vi "Make Panel Draggable - Drop In.vi"(0 "User Event":refnum<user-event>, 11 "error in (no error)":errorcluster) -> (15 "error out":errorcluster)   [LabVIEW 2011]
uses:
  <vilib>/Utility/inputDevices.llb/mouseAcquire.vi
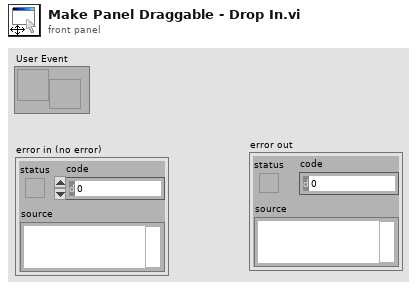
[diagram p1: front panel]
types:
  T1 = cluster{"Event Registration Refnum":refnum<event-registration>, "Event Registration Refnum":refnum<event-registration>}
  T2 = cluster{"Horizontal":i32, "Vertical":i32, "Scrolling":i32}
  T3 = typedef "LVRectTypeDef.ctl" = cluster{"left":i16, "top":i16, "right":i16, "bottom":i16}
  T4 = cluster{"button 1":bool, "button 2":bool, "button 3":bool, "button 4":bool}
  T5 = cluster{"Horizontal":i32, "Vertical":i32, "Horizontal":i32, "Vertical":i32}
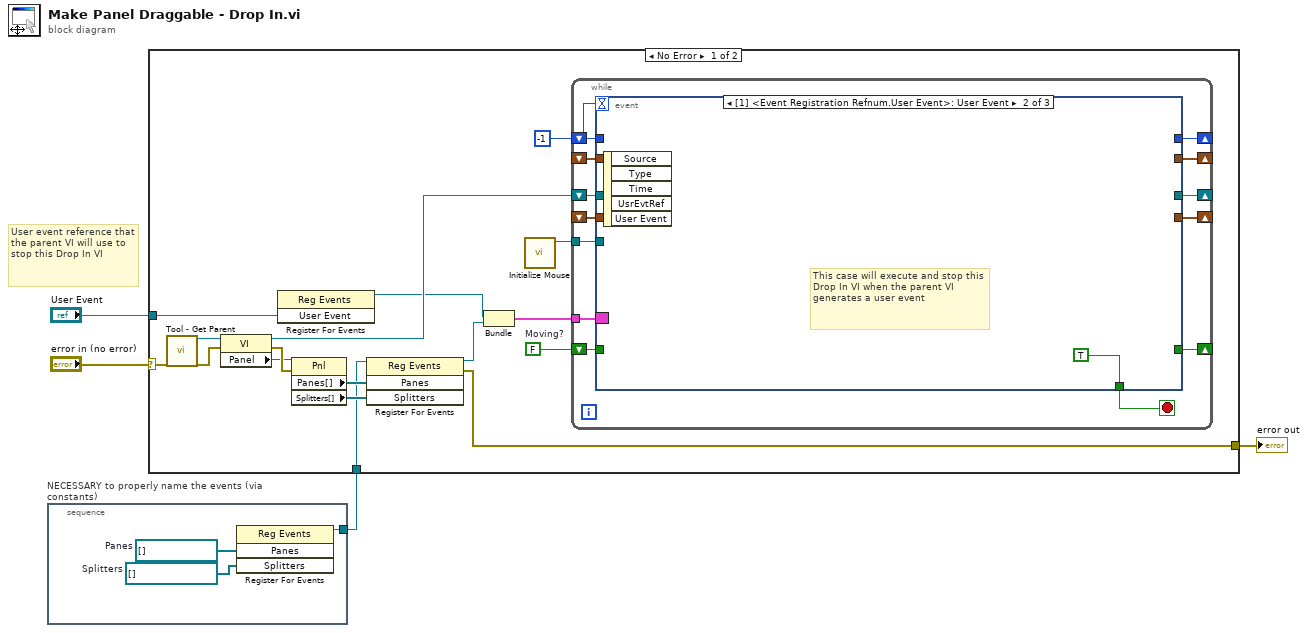
[diagram p0: block diagram]
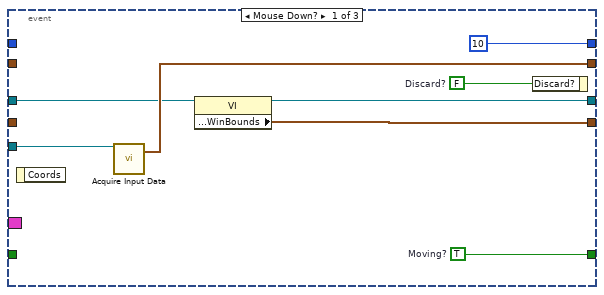
[diagram p2: hidden frame]
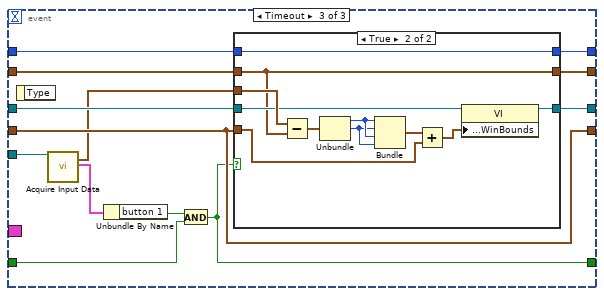
[diagram p3: hidden frame]
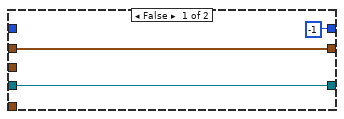
[diagram p4: hidden frame]
diagram:
  # "User event reference that the parent VI will use to stop this Drop In VI"
  n1 = stacked-sequence "NECESSARY to properly name the events (via constants)" {
    tunnel: [w5] -> w3
    frame #0 {
      w6 = refnum<vi>[] []  # Splitters
      w7 = refnum<vi>[] []  # Panes
      n2 = register-events(w7, w6) -> (reference out=w5:refnum<event-registration>)  [unwired: 2 in, 1 out]
    }
  }
  n3 = case shown="No Error" "error in (no error)" {
    selector: "error in (no error)" -> [w10 w74]
    tunnel: [w24 w74] -> w4
    tunnel: w3 -> [w11 _]
    tunnel: "User Event" -> [w9 _]
    frame No Error {
      w12 = FALSE  # Moving?
      n4 = call "Tool - Get Parent.vi"("error in (no error)"=w10) -> ("VI Refnum"=w16:refnum<vi>, "error out"=w21:errorcluster)  [unwired: 16 in, 1 out]
      n5 = property class="VI"(reference=w16, error in=w21) -> (reference out=w23:refnum<vi>, error out=w22:errorcluster, "Panel"=w17:refnum<vi>)
      n6 = register-events(w9) -> (reference out=w8:refnum<event-registration>)  [unwired: 2 in, 1 out]
      n7 = property class="Pnl"(reference=w17, error in=w22) -> ("Panes[]"=w18:refnum<vi>[], "Splitters[]"=w19:refnum<vi>[])  [unwired: 2 out]
      n8 = register-events(reference=w11, w18, w19) -> (reference out=w20:refnum<event-registration>, error out=w24:errorcluster)  [unwired: 1 in]
      n9 = Bundle("Event Registration Refnum"=w8, "Event Registration Refnum"=w20) -> (w15:T1)  [unwired: 1 out]
      n10 = call <vilib>:"Initialize Mouse.vi"() -> ("device ID"=w13:refnum<k1>)  [unwired: 1 in, 10 out]
      n11 = while {
        shift-right: [w37] -> _
        shift-left: _ -> [w34]
        shift-right: [w36] -> _
        shift-left: w12 -> [w35]
        shift-right: [w33] -> _
        shift-left: _ -> [w32]
        shift-right: [w31] -> _
        shift-left: w23 -> [w30]
        tunnel: w13 -> [w29]
        shift-right: [w28] -> _
        shift-left: -1 -> [w27]
        tunnel: w15 -> [w26]
        stop <- w25 stop-if-true
        n12 = event shown="[1] <Event Registration Refnum.User Event>: User Event" {
          selector: w26 -> [_ _ _]
          dyn-events: _ -> [_ _ _]
          timeout: w27 -> [_ _ _]
          tunnel: [w44 _ w59] -> w37
          tunnel: [w43 _ w48] -> w36
          tunnel: w35 -> [_ _ w49]
          tunnel: w34 -> [_ _ w59]
          tunnel: [w40 _ w47] -> w33
          tunnel: w32 -> [_ _ w57]
          tunnel: [w42 _ w51] -> w31
          tunnel: w30 -> [w38 _ w58]
          tunnel: w29 -> [w41 _ w56]
          tunnel: [10 _ w53] -> w28
          tunnel: w27 -> [_ _ w52]
          tunnel: [_ TRUE _] -> w25
          event Mouse Down? {
            w43 = TRUE  # Moving?
            w45 = FALSE  # Discard?
            n13 = event-data() -> ()  [unwired: 2 out]
            n14 = call-poly <vilib>:"Acquire Input Data.vi"("device ID"=w41) -> ("axis info"=w40:T2)  [unwired: 2 in, 16 out]
            n15 = property class="VI"(reference=w38) -> (reference out=w42:refnum<vi>, "Front Panel.WinBounds"=w44:T3)  [unwired: 1 in, 1 out]
            n16 = event-data("Discard?"=w45) -> ()  [unwired: 1 in, 1 out]
          }
          event User Event {
            # "This case will execute and stop this Drop In VI when the parent VI generates a user event"
            n17 = event-data() -> ()  [unwired: 6 out]
          }
          event Timeout {
            n18 = event-data() -> ()  [unwired: 2 out]
            n19 = call-poly <vilib>:"Acquire Input Data.vi"("device ID"=w56) -> ("axis info"=w55:T2, "button info"=w54:T4)  [unwired: 2 in, 15 out]
            n20 = Unbundle By Name(w54) -> ("button 1"=w50:bool)
            n21 = And(x=w50, y=w49) -> (x .and. y?=w48:bool)
            n22 = case shown="True" w48 {
              tunnel: w57 -> [w60 w63]
              tunnel: w55 -> [_ w73]
              tunnel: w59 -> [_ w69]
              tunnel: w58 -> [w61 w68]
              tunnel: [-1 w65] -> w53
              tunnel: w52 -> [_ w65]
              tunnel: [w61 w64] -> w51
              tunnel: [w60 w63] -> w47
              frame False {
              }
              frame True {
                n23 = Subtract(x=w73, y=w63) -> (x-y=w66:T2)
                n24 = Unbundle(w66) -> ("Horizontal"=w72:i32, "Vertical"=w71:i32)  [unwired: 1 out]
                n25 = Bundle("Horizontal"=w72, "Vertical"=w71, "Horizontal"=w72, "Vertical"=w71) -> (w70:T5)  [unwired: 1 out]
                n26 = Add(x=w70, y=w69) -> (x+y=w67:cluster{i32, i32, i32, i32})
                n27 = property class="VI"(reference=w68, "Front Panel.WinBounds"=w67) -> (reference out=w64:refnum<vi>)  [unwired: 1 in, 1 out]
              }
            }
          }
        }
      }
    }
    frame Error {
    }
  }
  "error out" <- w4
